vi "Timer FGV.vi"(7 "Action":T1, 8 "error in (no error)":errorcluster) -> (0 "error out":errorcluster, 3 "Elapsed Time":dbl)   [LabVIEW 2015]
uses:
  Timer Actions.ctl
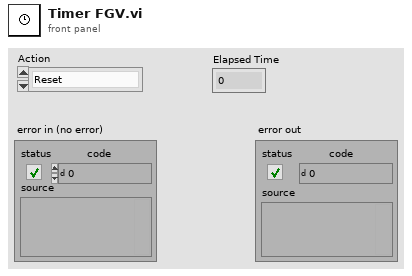
[diagram p1: front panel]
types:
  T1 = typedef "Timer Actions.ctl" = enum16{"Reset", "Get"}
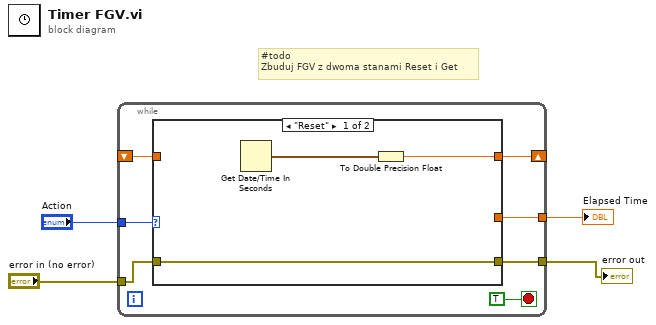
[diagram p0: block diagram]
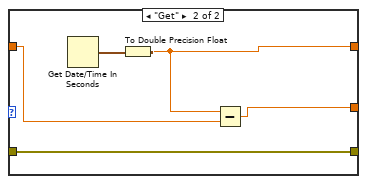
[diagram p2: hidden frame]
diagram:
  # "#todo \nZbuduj FGV z dwoma stanami Reset i Get"
  n1 = while {
    shift-right: [w8] -> _
    shift-left: _ -> [w9]
    tunnel: "Action" -> [w10]
    tunnel: "error in (no error)" -> [w6]
    tunnel: [w7] -> w2
    tunnel: [w5] -> w1
    stop <- TRUE stop-if-true
    n2 = case shown="\"Reset\"" w10 {
      tunnel: w9 -> [_ w18]
      tunnel: [w13 w17] -> w8
      tunnel: [_ w16] -> w7
      tunnel: w6 -> [w12 w15]
      tunnel: [w12 w15] -> w5
      frame "Reset" {
        n3 = Get Date/Time In Seconds() -> (seconds since 1Jan1904=w14:timestamp)
        n4 = To Double Precision Float(number=w14) -> (double precision float=w13:dbl)
      }
      frame "Get" {
        n5 = Get Date/Time In Seconds() -> (seconds since 1Jan1904=w19:timestamp)
        n6 = To Double Precision Float(number=w19) -> (double precision float=w17:dbl)
        n7 = Subtract(x=w17, y=w18) -> (x-y=w16:dbl)
      }
    }
  }
  "Elapsed Time" <- w2
  "error out" <- w1
